vi "RaceGame.vi"() -> ()   [LabVIEW 2013]
panel:
  out "P2_Win":bool
  out "P1_Wins":bool
  out "PC_2":dbl
  out "PC_1":dbl
  in  "P2":bool
  in  "P1":bool
  out "Carrera":bool
  out "P2_3":bool
  out "P2_2":bool
  out "P2_1":bool
  out "P1_3":bool
  out "P1_2":bool
  out "P1_1":bool
  out "P2_0":bool
  out "P1_0":bool
  in  "stop":bool
  in  "Start":bool
  out "Rojo":bool
  out "Amarillo2":bool
  out "Verde":bool
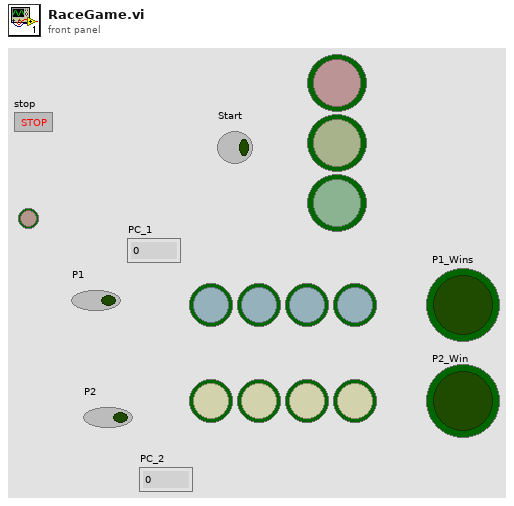
[diagram p1: front panel]
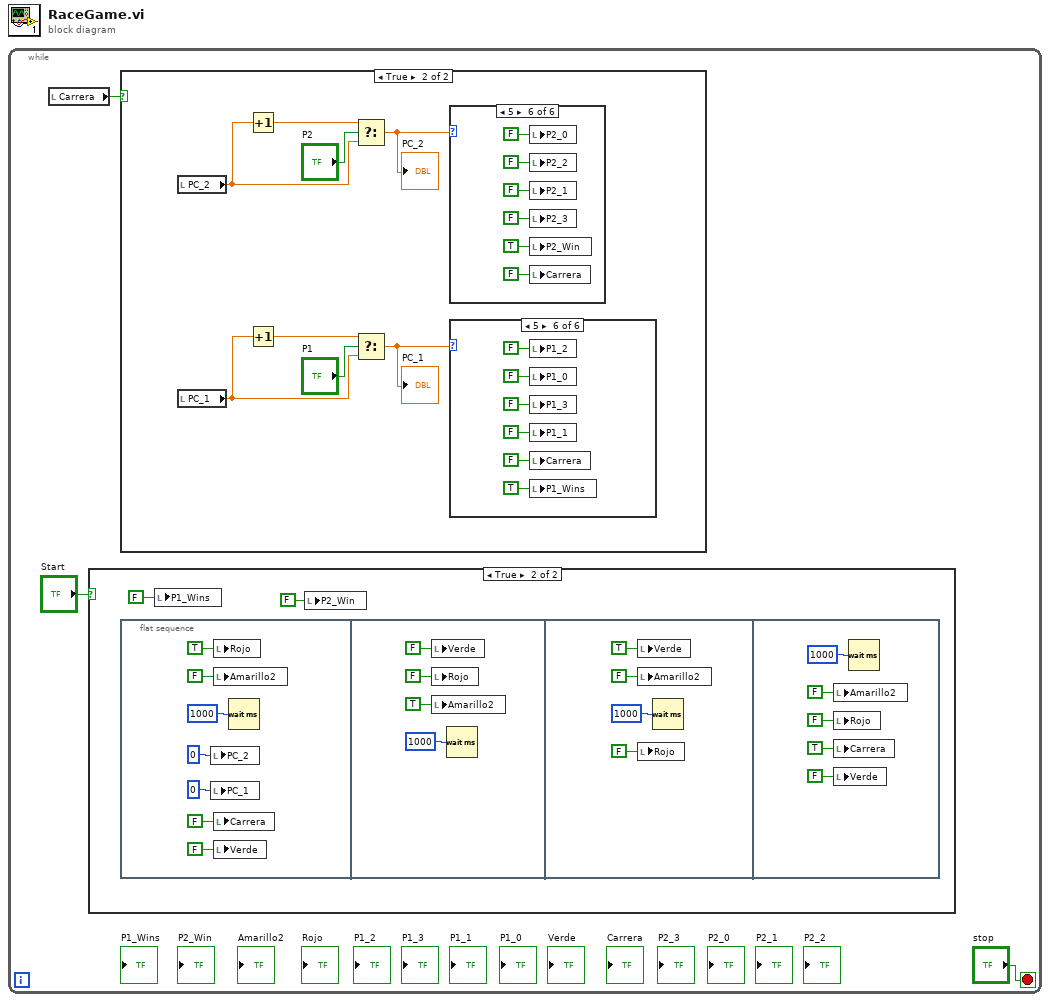
[diagram p0: block diagram]
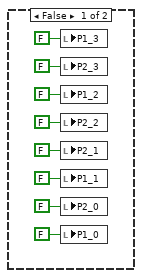
[diagram p2: hidden frame]
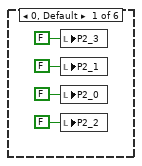
[diagram p3: hidden frame]
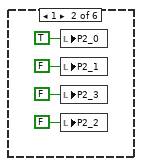
[diagram p4: hidden frame]
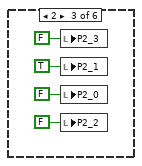
[diagram p5: hidden frame]
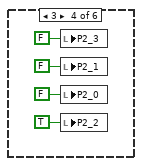
[diagram p6: hidden frame]
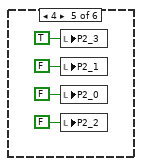
[diagram p7: hidden frame]
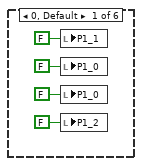
[diagram p8: hidden frame]
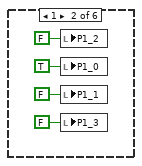
[diagram p9: hidden frame]
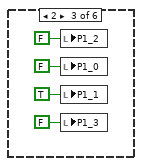
[diagram p10: hidden frame]
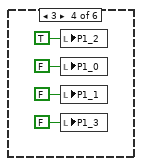
[diagram p11: hidden frame]
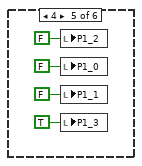
[diagram p12: hidden frame]
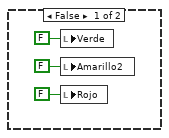
[diagram p13: hidden frame]
diagram:
  n1 = while {
    stop <- "stop" stop-if-true
    n2 = local read "Carrera"() -> (w1:bool)
    n3 = case shown="True" "Start" {
      frame False {
        n4 = local write "Verde"(FALSE ("Verde")) -> ()
        n5 = local write "Amarillo2"(FALSE ("Amarillo2")) -> ()
        n6 = local write "Rojo"(FALSE ("Rojo")) -> ()
      }
      frame True {
        n7 = flat-sequence {
          frame #0 {
            n8 = local write "PC_2"(0) -> ()
            n9 = local write "PC_1"(0) -> ()
            n10 = local write "Rojo"(TRUE ("Rojo")) -> ()
            n11 = local write "Amarillo2"(FALSE ("Amarillo2")) -> ()
            n12 = local write "Carrera"(FALSE ("Carrera")) -> ()
            n13 = local write "Verde"(FALSE ("Verde")) -> ()
            n14 = Wait (ms)(milliseconds to wait=u32 1000 ("millisecond timer value")) -> ()  [unwired: 1 out]
          }
          frame #1 {
            n15 = local write "Verde"(FALSE ("Verde")) -> ()
            n16 = local write "Rojo"(FALSE ("Rojo")) -> ()
            n17 = local write "Amarillo2"(TRUE ("Amarillo2")) -> ()
            n18 = Wait (ms)(milliseconds to wait=u32 1000 ("millisecond timer value")) -> ()  [unwired: 1 out]
          }
          frame #2 {
            n19 = local write "Verde"(TRUE ("Verde")) -> ()
            n20 = local write "Amarillo2"(FALSE ("Amarillo2")) -> ()
            n21 = local write "Rojo"(FALSE ("Rojo")) -> ()
            n22 = Wait (ms)(milliseconds to wait=u32 1000 ("millisecond timer value")) -> ()  [unwired: 1 out]
          }
          frame #3 {
            n23 = local write "Amarillo2"(FALSE ("Amarillo2")) -> ()
            n24 = local write "Rojo"(FALSE ("Rojo")) -> ()
            n25 = local write "Carrera"(TRUE ("Carrera")) -> ()
            n26 = local write "Verde"(FALSE ("Verde")) -> ()
            n27 = Wait (ms)(milliseconds to wait=u32 1000 ("millisecond timer value")) -> ()  [unwired: 1 out]
          }
        }
        n28 = local write "P1_Wins"(FALSE ("P1_Wins")) -> ()
        n29 = local write "P2_Win"(FALSE ("P2_Win")) -> ()
      }
    }
    n30 = case shown="True" w1 {
      frame False {
        n31 = local write "P1_3"(FALSE ("P1_3")) -> ()
        n32 = local write "P2_3"(FALSE ("P2_3")) -> ()
        n33 = local write "P1_2"(FALSE ("P1_2")) -> ()
        n34 = local write "P2_2"(FALSE ("P2_2")) -> ()
        n35 = local write "P2_1"(FALSE ("P2_1")) -> ()
        n36 = local write "P1_1"(FALSE ("P2_0")) -> ()
        n37 = local write "P2_0"(FALSE ("P2_0")) -> ()
        n38 = local write "P1_0"(FALSE ("P1_0")) -> ()
      }
      frame True {
        n39 = local read "PC_2"() -> (w14:dbl)
        n40 = local read "PC_1"() -> (w13:dbl)
        n41 = Increment(x=w14) -> (x+1=w15:dbl)
        n42 = Increment(x=w13) -> (x+1=w18:dbl)
        n43 = Select(t=w15, s="P2", f=w14) -> (s? t:f=w17:dbl)
        "PC_2" <- w17
        n44 = Select(t=w18, s="P1", f=w13) -> (s? t:f=w12:dbl)
        "PC_1" <- w12
        n45 = case shown="5" w17 {
          frame 0, Default {
            n46 = local write "P2_3"(FALSE ("Verde")) -> ()
            n47 = local write "P2_1"(FALSE ("Verde")) -> ()
            n48 = local write "P2_0"(FALSE ("Verde")) -> ()
            n49 = local write "P2_2"(FALSE ("Verde")) -> ()
          }
          frame 1 {
            n50 = local write "P2_0"(TRUE ("Verde")) -> ()
            n51 = local write "P2_1"(FALSE ("Verde")) -> ()
            n52 = local write "P2_3"(FALSE ("Verde")) -> ()
            n53 = local write "P2_2"(FALSE ("Verde")) -> ()
          }
          frame 2 {
            n54 = local write "P2_3"(FALSE ("Verde")) -> ()
            n55 = local write "P2_1"(TRUE ("Verde")) -> ()
            n56 = local write "P2_0"(FALSE ("Verde")) -> ()
            n57 = local write "P2_2"(FALSE ("Verde")) -> ()
          }
          frame 3 {
            n58 = local write "P2_3"(FALSE ("Verde")) -> ()
            n59 = local write "P2_1"(FALSE ("Verde")) -> ()
            n60 = local write "P2_0"(FALSE ("Verde")) -> ()
            n61 = local write "P2_2"(TRUE ("Verde")) -> ()
          }
          frame 4 {
            n62 = local write "P2_3"(TRUE ("Verde")) -> ()
            n63 = local write "P2_1"(FALSE ("Verde")) -> ()
            n64 = local write "P2_0"(FALSE ("Verde")) -> ()
            n65 = local write "P2_2"(FALSE ("Verde")) -> ()
          }
          frame 5 {
            n66 = local write "P2_0"(FALSE ("P2_0")) -> ()
            n67 = local write "P2_2"(FALSE ("P2_2")) -> ()
            n68 = local write "P2_1"(FALSE ("P2_1")) -> ()
            n69 = local write "P2_3"(FALSE ("P2_3")) -> ()
            n70 = local write "P2_Win"(TRUE ("P2_Win")) -> ()
            n71 = local write "Carrera"(FALSE ("Carrera")) -> ()
          }
        }
        n72 = case shown="5" w12 {
          frame 0, Default {
            n73 = local write "P1_1"(FALSE ("Verde")) -> ()
            n74 = local write "P1_0"(FALSE ("Verde")) -> ()
            n75 = local write "P1_0"(FALSE ("Verde")) -> ()
            n76 = local write "P1_2"(FALSE ("Verde")) -> ()
          }
          frame 1 {
            n77 = local write "P1_2"(FALSE ("Verde")) -> ()
            n78 = local write "P1_0"(TRUE ("Verde")) -> ()
            n79 = local write "P1_1"(FALSE ("Verde")) -> ()
            n80 = local write "P1_3"(FALSE ("Verde")) -> ()
          }
          frame 2 {
            n81 = local write "P1_2"(FALSE ("Verde")) -> ()
            n82 = local write "P1_0"(FALSE ("Verde")) -> ()
            n83 = local write "P1_1"(TRUE ("Verde")) -> ()
            n84 = local write "P1_3"(FALSE ("Verde")) -> ()
          }
          frame 3 {
            n85 = local write "P1_2"(TRUE ("Verde")) -> ()
            n86 = local write "P1_0"(FALSE ("Verde")) -> ()
            n87 = local write "P1_1"(FALSE ("Verde")) -> ()
            n88 = local write "P1_3"(FALSE ("Verde")) -> ()
          }
          frame 4 {
            n89 = local write "P1_2"(FALSE ("Verde")) -> ()
            n90 = local write "P1_0"(FALSE ("Verde")) -> ()
            n91 = local write "P1_1"(FALSE ("Verde")) -> ()
            n92 = local write "P1_3"(TRUE ("Verde")) -> ()
          }
          frame 5 {
            n93 = local write "P1_2"(FALSE ("P1_2")) -> ()
            n94 = local write "P1_0"(FALSE ("P1_0")) -> ()
            n95 = local write "P1_3"(FALSE ("P1_3")) -> ()
            n96 = local write "P1_1"(FALSE ("P1_1")) -> ()
            n97 = local write "Carrera"(FALSE ("Carrera")) -> ()
            n98 = local write "P1_Wins"(TRUE ("P1_Wins")) -> ()
          }
        }
      }
    }
  }
